vi "RGB_set.vi"(2 "error in":errorcluster, 3 "RGB":u16[](array[numeric]), 4 "Channel_start":u8, 5 "SCI":u8) -> (0 "error out":errorcluster)   [LabVIEW 2013]
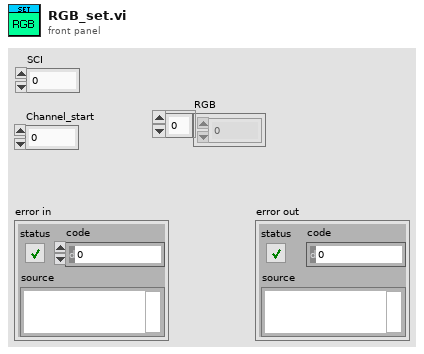
[diagram p1: front panel]
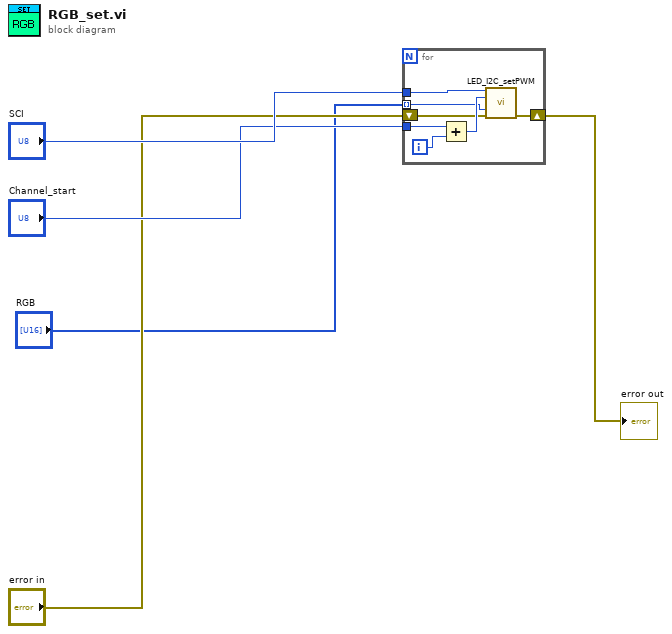
[diagram p0: block diagram]
diagram:
  n1 = for {
    tunnel: "SCI" -> [w12]
    tunnel: "Channel_start" -> [w11]
    shift-right: [w8] -> w2
    shift-left: "error in" -> [w7]
    tunnel: "RGB" -> [w6] mode=indexing
    i -> [w10]
    n2 = Add(x=w11, y=w10) -> (x+y=w9:i32)
    n3 = call "LED_I2C_setPWM.vi"("Servo Controller Index"=w12, "PWM Channel"=w9, "Off (duty-cycle)"=w6, "Error In"=w7) -> ("Error Out"=w8:errorcluster)  [unwired: 11 in]
  }
  "error out" <- w2
